vi "Main On Load Action VI.vi"(8 "error in (no error)":errorcluster, 11 "Device Item Ref in":T1 format="%.0x") -> (0 "error out":errorcluster, 3 "Device Item Ref out":T1 format="%.0x")   [LabVIEW 2015, in "AIT 429 System Explorer.lvlib"]
uses:
  AIT 429 System Explorer.lvlib
  <vilib>/NI Veristand/Custom Device API/Custom Device Item Ref.ctl
  <vilib>/NI Veristand/Custom Device API/Custom Device Path Data.ctl
  <vilib>/NI Veristand/Custom Device API/Custom Device Supported Target.ctl
  <vilib>/NI Veristand/Custom Device API/Path Specification.ctl
  <vilib>/NI Veristand/Custom Device API/Path Type.ctl
  <vilib>/NI Veristand/Custom Device API/Custom Device Execution Mode.ctl
  Shared/Controls and Global/Specify module by.ctl
  NationalInstruments.VeriStand.SystemDefinitionAPI
  Shared/Controls and Global/Global.vi
  <vilib>/NI Veristand/Custom Device API/Get Item Property (Variant).vi
  <vilib>/NI Veristand/Custom Device API/Set Item Property (Variant).vi
  <vilib>/NI Veristand/Custom Device API/Set Item Property (U16).vi
  <vilib>/NI VeriStand/Custom Device API/Custom Device API.lvlib
  Shared/ARINC 429 Shared.lvlib
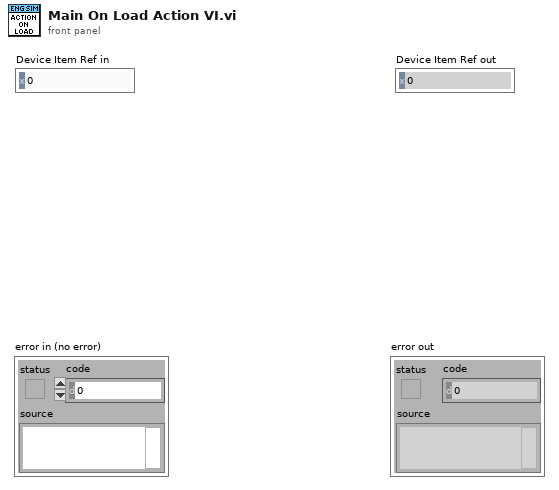
[diagram p1: front panel]
types:
  T1 = typedef "Custom Device API.lvlib/Custom Device Item Ref.ctl" = u64
  T2 = typedef "Custom Device API.lvlib/Path Specification.ctl" = cluster{"Path":path, "Type":T3}
  T3 = typedef "Custom Device API.lvlib/Path Type.ctl" = enum16{"Absolute", "To Base", "To Common Data Dir", "To Application Data Dir"}
  T4 = typedef "Custom Device API.lvlib/Custom Device Execution Mode.ctl" = enum16{"Asynchronous", "Inline HW Interface", "Inline Model Interface", "Inline Timing and Sync", "Asynchronous Timing and Sync"}
  T5 = typedef "Custom Device API.lvlib/Custom Device Supported Target.ctl" = enum16{"All", "PharLap", "VxWorks", "Windows", "Linux_32_ARM", "Linux_x64", "PharLap & Windows", "PharLap & VxWorks", "VxWorks & Windows"}
  T6 = typedef "Custom Device API.lvlib/Custom Device Path Data.ctl" = cluster{"SupportedTarget":T5, "Source":T2, "RT Destination":path}
  T7 = typedef "ARINC 429 Shared.lvlib/Specify module by.ctl" = enum16{"Index", "SlotID", "Serial number"}
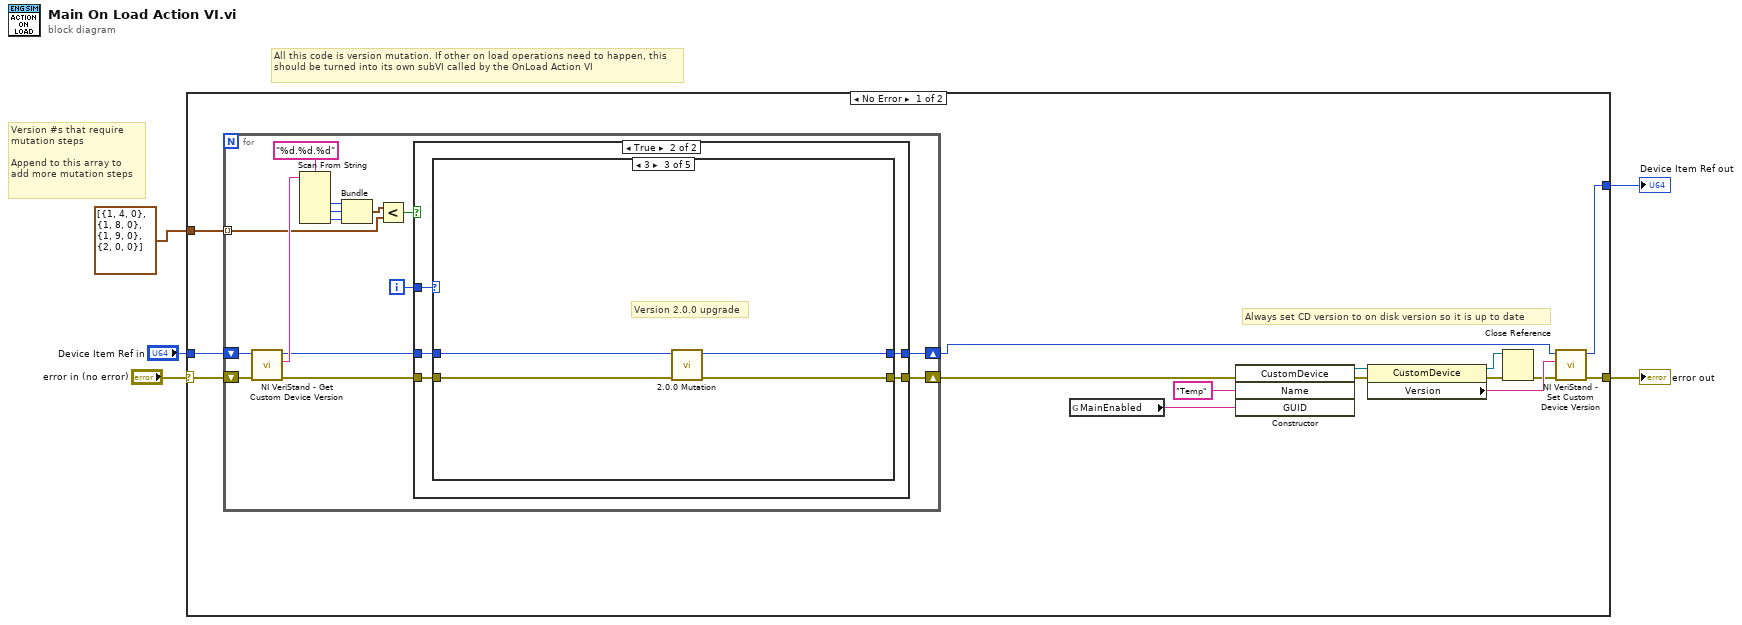
[diagram p0: block diagram]
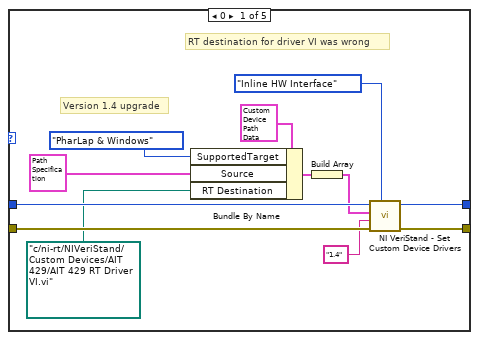
[diagram p3: hidden frame]
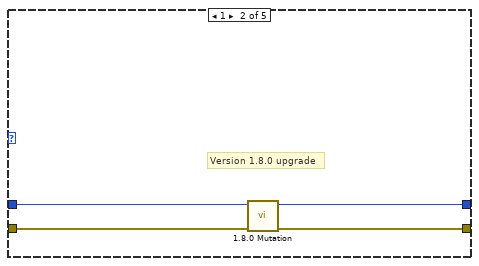
[diagram p4: hidden frame]
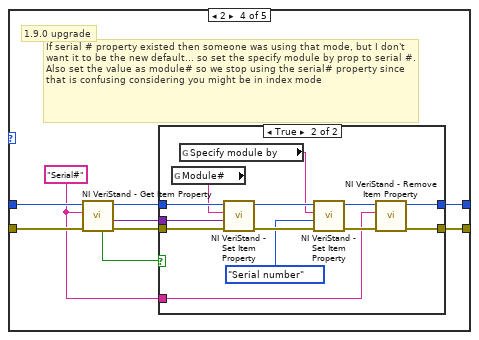
[diagram p5: hidden frame]
diagram:
  # "All this code is version mutation. If other on load operations need to happen, this should be turned into its own subVI called by the OnLoad Action VI"
  # "Version #s that require\nmutation steps\n\nAppend to this array to\nadd more mutation steps"
  n1 = case shown="No Error" "error in (no error)" {
    selector: "error in (no error)" -> [w19 w90]
    tunnel: [w8 w90] -> w4
    tunnel: "Device Item Ref in" -> [w18 w89]
    tunnel: [w7 w89] -> w2
    tunnel: cluster{i32, i32, i32}[] [{1, 4, 0}, {1, 8, 0}, {1, 9, 0}, {2, 0, 0}] -> [w20 _]
    frame No Error {
      # "Always set CD version to on disk version so it is up to date"
      n2 = for {
        tunnel: w20 -> [w22] mode=indexing
        shift-right: [w26] -> w16
        shift-left: w19 -> [w31]
        shift-right: [w24] -> w17
        shift-left: w18 -> [w30]
        i -> [w23]
        n3 = call <vilib>:"NI VeriStand - Get Custom Device Version.vi"("error in (no error)"=w31, "Device Ref in"=w30) -> ("error out"=w27:errorcluster, "Value"=w29:string, "Device Ref out"=w25:T1)  [unwired: 7 in]
        n4 = Scan From String(format string="%d.%d.%d", input string=w29) -> (output 1=w33:i32, output 2=w34:i32, output 3=w21:i32)  [unwired: 5 in, 3 out]
        n5 = Bundle(w33, w34, w21) -> (w35:cluster{i32, i32, i32})  [unwired: 1 in]
        n6 = Less?(x=w35, y=w22) -> (x < y?=w28:bool)
        n7 = case shown="True" w28 {
          tunnel: w27 -> [w37 w42]
          tunnel: [w37 w41] -> w26
          tunnel: w25 -> [w36 w38]
          tunnel: [w36 w39] -> w24
          tunnel: w23 -> [_ w40]
          frame False {
          }
          frame True {
            n8 = case shown="3" w40 {
              tunnel: w42 -> [w52 w58 w62 w71 w88]
              tunnel: [w44 w56 w60 w65 w88] -> w41
              tunnel: [w54 w55 w59 w64 w87] -> w39
              tunnel: w38 -> [w51 w57 w61 w70 w87]
              frame 0 {
                # "RT destination for driver VI was wrong"
                # "Version 1.4 upgrade"
                n9 = Bundle By Name(cluster=T6 {"SupportedTarget"=enum."All", "Source"={"Path"=path "", "Type"=enum."Absolute"}, "RT Destination"=path ""} ("Driver VI Path"), "SupportedTarget"=Custom_Device_Supported_Target."PharLap & Windows", "Source"=T2 {"Path"=path "Custom Devices/AIT 429/AIT 429 RT Driver VI.vi", "Type"=enum."To Common Data Dir"}, "RT Destination"=path "c:/ni-rt/NIVeriStand/Custom Devices/AIT 429/AIT 429 RT Driver VI.vi") -> (w49:T6)
                n10 = Build Array(w49) -> (w48:T6[])
                n11 = call <vilib>:"NI VeriStand - Set Custom Device Drivers.vi"("Execution mode"=Custom_Device_Execution_Mode."Inline HW Interface", "error in (no error)"=w52, "Version"="1.4" ("format string"), "Driver VI"=w48, "Device Ref in"=w51) -> ("error out"=w44:errorcluster, "Device Ref out"=w54:T1)  [unwired: 5 in]
              }
              frame 1 {
                # "Version 1.8.0 upgrade"
                n12 = call "1.8.0 Mutation.vi"("error in"=w58, "Device Ref in"=w57) -> ("error out"=w56:errorcluster, "Device Ref out"=w55:T1)  [unwired: 8 in]
              }
              frame 3 {
                # "Version 2.0.0 upgrade"
                n13 = call "2.0.0 Mutation.vi"("error in"=w62, "Device Ref in"=w61) -> ("error out"=w60:errorcluster, "Device Ref out"=w59:T1)  [unwired: 8 in]
              }
              frame 2 {
                w63 = "Serial#" ("x")
                # "If serial # property existed then someone was using that mode, but I don't want it to be the new default... so set the specify module by prop to serial #. Also set the value as module# so we stop using the serial# property since that is confusing considering you might be in index mode"
                # "1.9.0 upgrade"
                n14 = call-poly <vilib>:"NI VeriStand - Get Item Property.vi"("error in (no error)"=w71, "Property Name"=w63, "Item Ref in"=w70) -> ("error out"=w68:errorcluster, "Value"=w66:variant, "Item Ref out"=w67:T1, "Found?"=w69:bool)  [unwired: 5 in]
                n15 = case shown="True" w69 {
                  tunnel: w68 -> [w72 w86]
                  tunnel: w67 -> [w73 w85]
                  tunnel: w66 -> [_ w83]
                  tunnel: [w72 w77] -> w65
                  tunnel: [w73 w75] -> w64
                  tunnel: w63 -> [_ w74]
                  frame False {
                  }
                  frame True {
                    n16 = global read "Global.vi" "Module#"() -> (w84:string)
                    n17 = global read "Global.vi" "Specify module by"() -> (w80:string)
                    n18 = call-poly <vilib>:"NI VeriStand - Set Item Property.vi"("error in (no error)"=w86, "Value"=w83, "Property Name"=w84, "Item Ref in"=w85) -> ("error out"=w81:errorcluster, "Item Ref out"=w82:T1)  [unwired: 5 in, 1 out]
                    n19 = call-poly <vilib>:"NI VeriStand - Set Item Property.vi"("error in (no error)"=w81, "Value"=Specify_module_by."Serial number" ("Specify module by"), "Property Name"=w80, "Item Ref in"=w82) -> ("error out"=w78:errorcluster, "Item Ref out"=w76:T1)  [unwired: 5 in, 1 out]
                    n20 = call <vilib>:"NI VeriStand - Remove Item Property.vi"("error in (no error)"=w78, "Property Name"=w74, "Item Ref in"=w76) -> ("error out"=w77:errorcluster, "Item Ref out"=w75:T1)  [unwired: 6 in, 1 out]
                  }
                }
              }
              frame Default {
              }
            }
          }
        }
      }
      n21 = global read "Global.vi" "MainEnabled"() -> (w6:string)
      n22 = constructor class="CustomDevice"(error in=w16, "Name"="Temp", "GUID"=w6) -> (reference out=w14:refnum<k24>, error out=w13:errorcluster)  [unwired: 2 in, 3 out]
      n23 = property class="CustomDevice"(reference=w14, error in=w13) -> (reference out=w11:refnum<k24>, error out=w12:errorcluster, "Version"=w10:string)
      n24 = Close Reference(reference=w11, error in (no error)=w12) -> (error out=w9:errorcluster)
      n25 = call <vilib>:"NI VeriStand - Set Custom Device Version.vi"("error in (no error)"=w9, "Value"=w10, "Device Ref in"=w17) -> ("error out"=w8:errorcluster, "Device Ref out"=w7:T1)  [unwired: 7 in]
    }
    frame Error {
    }
  }
  "error out" <- w4
  "Device Item Ref out" <- w2
